vi "Read passerId.vi"(8 "error in (no error)":errorcluster, 11 "PositionTactic in":refnum<class "PositionTactic.lvclass">) -> (0 "error out":errorcluster, 2 "passerId":u8, 3 "PositionTactic out":refnum<class "PositionTactic.lvclass">)   [LabVIEW 2023, in "PositionTactic.lvclass"]
uses:
  PositionTactic.lvclass
  PositionTactic.lvclass/PositionTactic.ctl
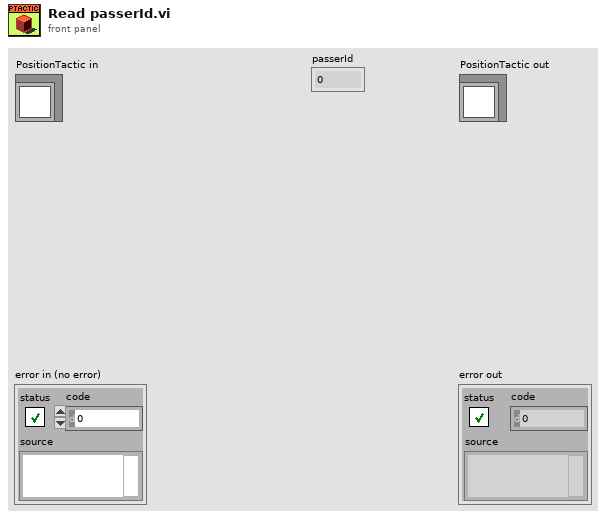
[diagram p1: front panel]
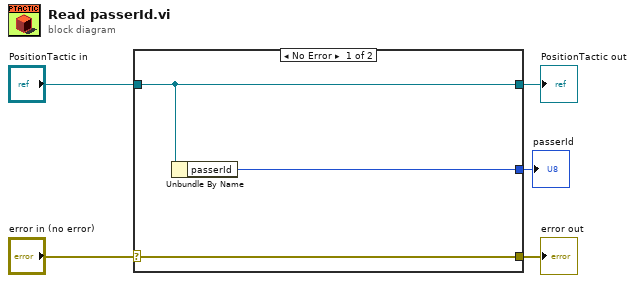
[diagram p0: block diagram]
diagram:
  n1 = case shown="No Error" "error in (no error)" {
    selector: "error in (no error)" -> [w8 w9]
    tunnel: [w8 w9] -> w4
    tunnel: [w7 w10] -> w2
    tunnel: "PositionTactic in" -> [w7 w10]
    tunnel: [w6 _] -> w1
    frame No Error {
      n2 = Unbundle By Name(w7) -> ("passerId"=w6:u8)
    }
    frame Error {
    }
  }
  "error out" <- w4
  "PositionTactic out" <- w2
  "passerId" <- w1
